vi "Class to Variant.vi"(8 "error in (no error)":errorcluster, 10 "Data in":variant, 11 "VIP Publish Node in":refnum<class "VIP Publish Node.lvclass">) -> (0 "error out":errorcluster, 1 "Serialized Object Name":string, 2 "Data Out":variant, 3 "VIP Publish Node out":refnum<class "VIP Publish Node.lvclass">)   [LabVIEW 2014, in "VIP Publish Node.lvclass"]
uses:
  VIP Publish Node.lvclass
  Shared/Controls/VIP Publish - STYP.ctl
  VIP Publish Node.lvclass/VIP Publish Node.ctl
  Classes/Build Job/Build Job.lvclass
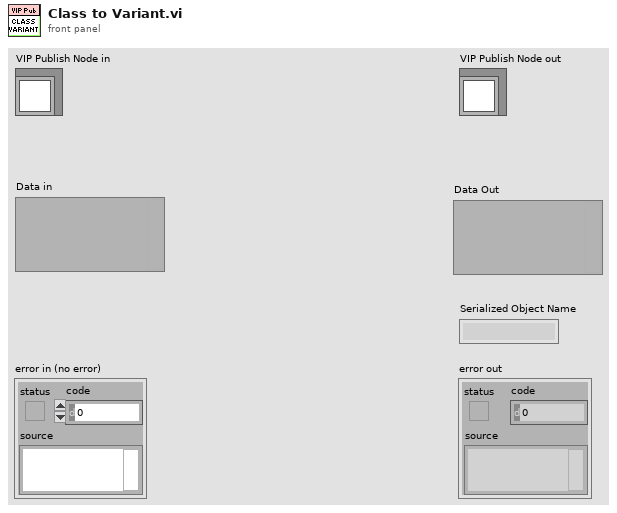
[diagram p1: front panel]
types:
  T1 = typedef "VIP Publish - STYP.ctl" = cluster{"VIP Path":string, "Repo Name":string}
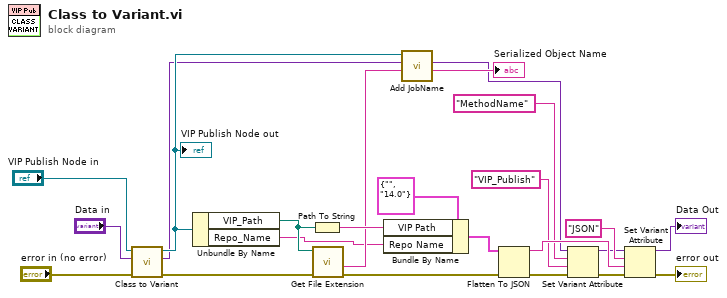
[diagram p0: block diagram]
diagram:
  n1 = call-parent "Class to Variant.vi"("error in (no error)"="error in (no error)", "Data in"="Data in", "Build Job in"="VIP Publish Node in") -> ("error out"=w6:errorcluster, "Data Out"=w3:variant, "Build Job out"=w8:refnum<class "VIP Publish Node.lvclass">)  [unwired: 5 in, 1 out]
  "VIP Publish Node out" <- w8
  n2 = Unbundle By Name(w8) -> ("VIP_Path"=w7:path, "Repo_Name"=w1:string)
  n3 = Path To String(path=w7) -> (string=w13:string)
  n4 = call <vilib>:"Get File Extension.vi"("error in (no error)"=w6, "file"=w7) -> ("error out"=w5:errorcluster, "filename without extension"=w9:string)  [unwired: 6 in, 2 out]
  n5 = Bundle By Name(cluster=T1 {"VIP Path"="", "Repo Name"="14.0"} ("VIPB Build"), "VIP Path"=w13, "Repo Name"=w1) -> (w15:T1)
  n6 = call "Add JobName.vi"("Job Target"=w9, "Data in"=w3, "Build Job in"=w8) -> ("Job Name"=→"Serialized Object Name":string, "Data Out"=w2:variant)  [unwired: 7 in]
  n7 = Flatten To JSON(anything=w15, error in (no error)=w5) -> (JSON string=w20:string, 11:w21:errorcluster)  [unwired: 1 in]
  n8 = Set Variant Attribute(Variant=w2, name="MethodName", value="VIP_Publish", error in=w21) -> (Variant out=w10:variant, error out=w16:errorcluster)  [unwired: 1 out]
  n9 = Set Variant Attribute(Variant=w10, name="JSON" ("Name"), value=w20, error in=w16) -> (Variant out=→"Data Out":variant, error out=→"error out":errorcluster)  [unwired: 1 out]
